vi "Config-Meas-Trigger.vi"(6 "manual step delay":dbl format="%^.2e", 7 "step delay\n(manual: 0)":u16(ring) items=["manual ->", "maximum", "minimum"], 8 "error in (no error)":errorcluster, 9 "polarity":bool, 10 "trigger function\n(disable: 0)":u16(ring), 11 "VISA session":refnum<visa-resource-name>) -> (0 "error out":errorcluster, 3 "VISA resource name out":refnum<visa-resource-name>)   [LabVIEW 2016, in "Agilent 415X Series.lvlib"]
doc: "This VI configures the trigger parameters for sweep/sampling measurement. \n\nThis VI does NOT actively check for errors, nor does it verify the measurement mode the instrument is currently in. Therefore it is the user's responsibility to make certain that Trigger Output mode is only used in SWEEP mode."
uses:
  Agilent 415X Series.lvlib
panel:
  # "(sec)"
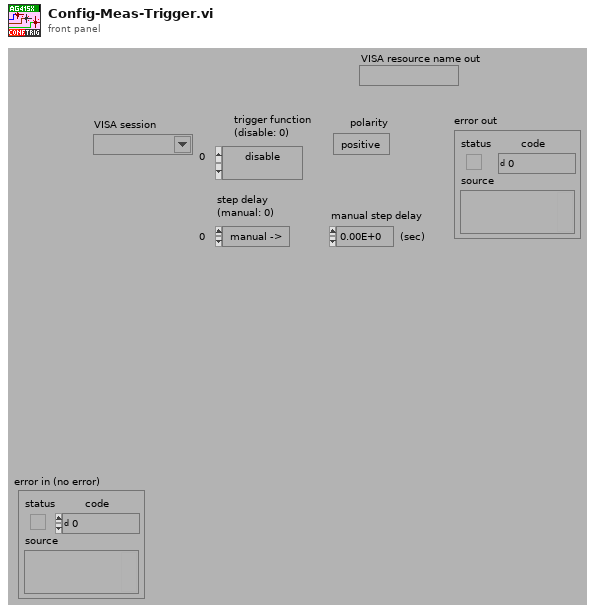
[diagram p1: front panel]
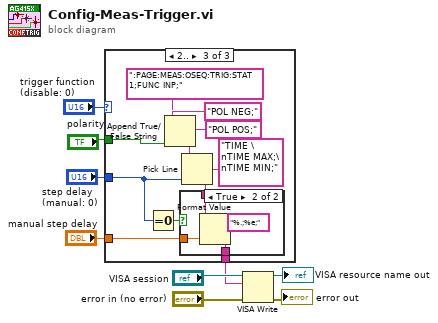
[diagram p0: block diagram]
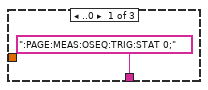
[diagram p2: hidden frame]
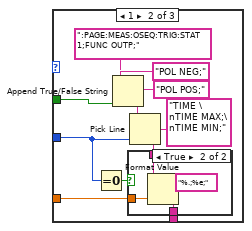
[diagram p3: hidden frame]
diagram:
  n1 = case shown="2.." "trigger function\n(disable: 0)" {
    tunnel: "polarity" -> [_ w21 w37]
    tunnel: "step delay\n(manual: 0)" -> [_ w16 w32]
    tunnel: "manual step delay" -> [_ w15 w31]
    tunnel: [":PAGE:MEAS:OSEQ:TRIG:STAT 0;" w12 w28] -> w2
    frame ..0 {
    }
    frame 1 {
      n2 = Equal To 0?(x=w16) -> (x = 0?=w11:bool)
      n3 = Append True/False String(1:w21, 2:"POL POS;", 3:"POL NEG;", 4:":PAGE:MEAS:OSEQ:TRIG:STAT 1;FUNC OUTP;") -> (0:w17:string)
      n4 = Pick Line(string ("")=w17, multi-line string="TIME \nTIME MAX;\nTIME MIN;", line index=w16) -> (output string=w13:string)
      n5 = case shown="True" w11 {
        tunnel: w15 -> [_ w25]
        tunnel: w13 -> [w22 w26]
        tunnel: [w22 w23] -> w12
        frame False {
        }
        frame True {
          n6 = Format Value(string ("")=w26, format string="%.;%e;", value (0)=w25) -> (output string=w23:string)
        }
      }
    }
    frame 2.. {
      n7 = Equal To 0?(x=w32) -> (x = 0?=w27:bool)
      n8 = Append True/False String(1:w37, 2:"POL POS;", 3:"POL NEG;", 4:":PAGE:MEAS:OSEQ:TRIG:STAT 1;FUNC INP;") -> (0:w33:string)
      n9 = Pick Line(string ("")=w33, multi-line string="TIME \nTIME MAX;\nTIME MIN;", line index=w32) -> (output string=w29:string)
      n10 = case shown="True" w27 {
        tunnel: w31 -> [_ w41]
        tunnel: w29 -> [w38 w42]
        tunnel: [w38 w39] -> w28
        frame False {
        }
        frame True {
          n11 = Format Value(string ("")=w42, format string="%.;%e;", value (0)=w41) -> (output string=w39:string)
        }
      }
    }
  }
  n12 = VISA Write(VISA resource name="VISA session", write buffer=w2, error in (no error)="error in (no error)") -> (VISA resource name out=→"VISA resource name out":refnum<visa-resource-name>, error out=→"error out":errorcluster)  [unwired: 1 out]
